vi "Adaptive Filter 2 Test.vi"(4 "Beta":fxp<+/-,32,-16>, 6 "Noise":T1, 7 "Filter Size":i32, 8 "Taps In":refnum<data-value>, 9 "Weights In":refnum<data-value>, 11 "Input":fxp<+/-,16,16>) -> (0 "Taps Out":refnum<data-value>, 1 "Weights Out":refnum<data-value>, 3 "Error Out":fxp<+/-,16,16> format="%.16g")   [LabVIEW 2016]
uses:
  <vilib>/Platform/TimedLoop/XDataNode/timing_clust.ctl
  <vilib>/Platform/TimedLoop/XDataNode/nitl_modes.ctl
  <vilib>/Platform/TimedLoop/XDataNode/wakeup.ctl
  <vilib>/Platform/TimedLoop/XDataNode/XDataNode.xnode
  <vilib>/Platform/TimedLoop/XDataNode/XDNodeRunTimeDep.lvlib
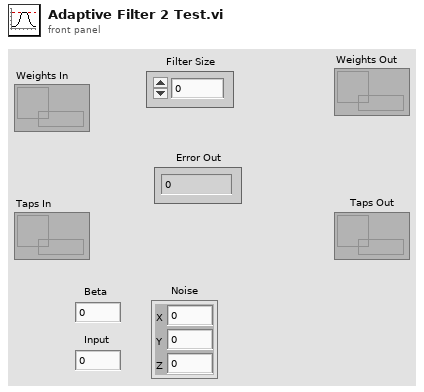
[diagram p1: front panel]
types:
  T1 = cluster{"X":fxp<+/-,16,16>, "Y":fxp<+/-,16,16>, "Z":fxp<+/-,16,16>}
  T2 = typedef "XDNodeRunTimeDep.lvlib/timing_clust.ctl" = cluster{"Expected End [f-1]":u64, "Actual End [f-1]":u64, "Finished Late? [f-1]":bool, "Expected End [i-1]":u64, "Actual End [i-1]":u64, "Finished Late? [i-1]":bool, "Expected Start [i]":u64, "Actual Start [i]":u64, "Expected Start [f]":u64, "Actual Start [f]":u64, "Source Name":string, "Structure Name":string, "Period":i64, "Deadline":i64, "Offset":i64, "Start":i64, "Priority":i32, "Timeout":i32, "Mode":T3, "Wakeup Reason":T4, "Error":errorcluster, "Source Type":string, "Secondary Source Type":string, "Global End Time":u64, "Global Start Time":u64, "Frame Duration":u64, "Iteration Duration":u64, "Assigned CPU":i32, "I/O Scan Engine Mode":u32}
  T3 = typedef "XDNodeRunTimeDep.lvlib/nitl_modes.ctl" = enum32{"No Change", "Process missed periods, maintain original phase", "Discard missed periods, maintain original phase", "Process missed periods, ignore original phase", "Discard missed periods, ignore original phase"}
  T4 = typedef "XDNodeRunTimeDep.lvlib/wakeup.ctl" = enum32{"Normal", "Aborted", "Asynchronous wakeup", "Timing source error", "Timed loop error", "Timeout"}
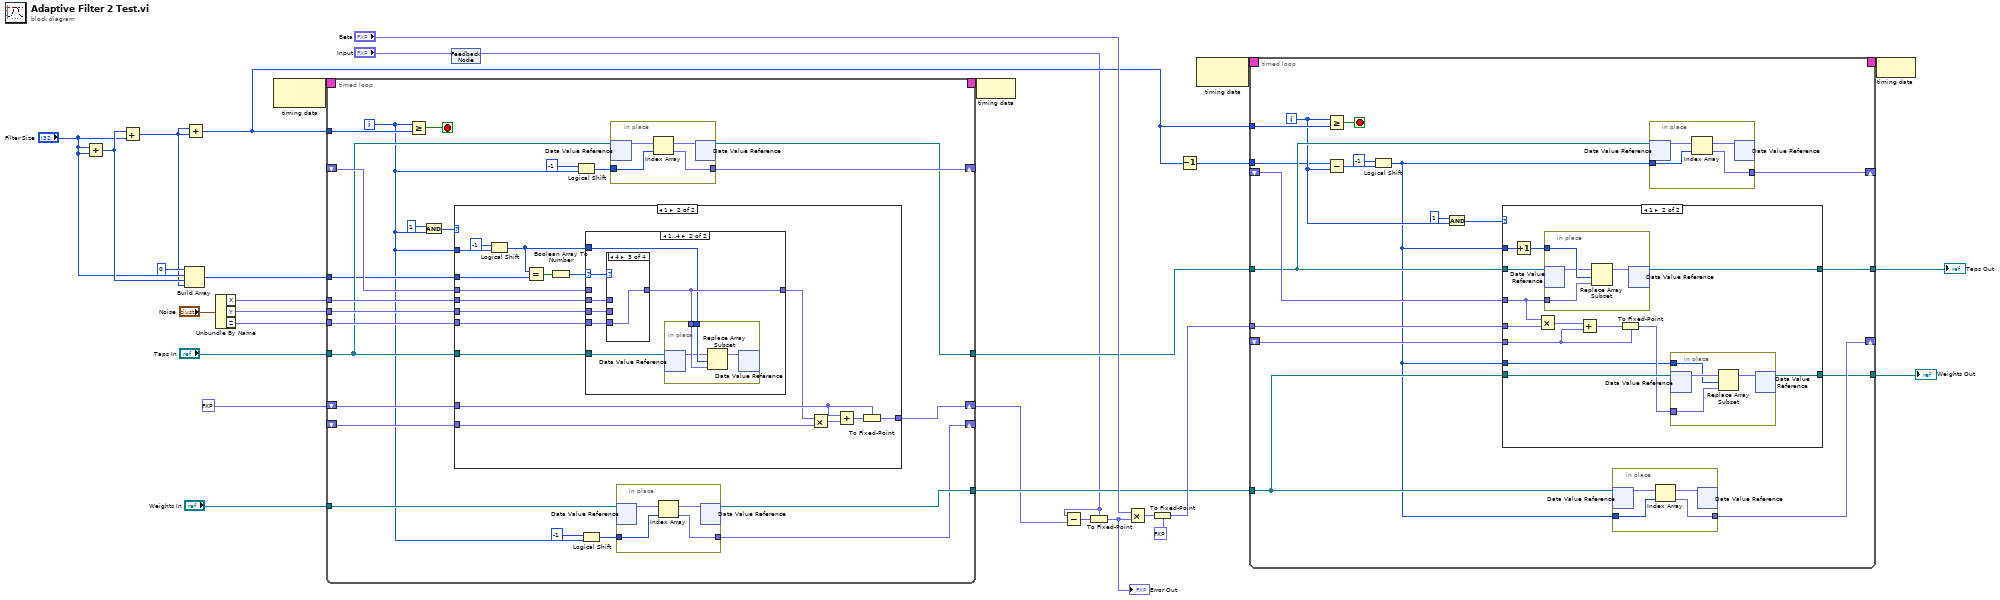
[diagram p0: block diagram]
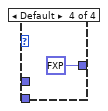
[diagram p7: hidden frame]
diagram:
  n1 = Add(x="Filter Size", y="Filter Size") -> (x+y=w12:i32)
  n2 = Add(x=w12, y="Filter Size") -> (x+y=w8:i32)
  n3 = Build Array(0 ("element"), "Filter Size", w12, w8) -> (w9:i32[])
  n4 = Add(x=w8, y=w8) -> (x+y=w6:i32)
  n5 = Unbundle By Name("Noise") -> ("X"=w30:fxp<+/-,16,16>, "Y"=w29:fxp<+/-,16,16>, "Z"=w28:fxp<+/-,16,16>)
  n6 = node-c288() -> (w24:T2)  [unwired: 1 in]
  n7 = timed-loop {
    tunnel: w30 -> [w40]
    tunnel: w29 -> [w39]
    tunnel: w28 -> [w38]
    shift-right: [w42] -> w14
    shift-left: fxp<+/-,33,19> 0.0 ("x+y") -> [w43]
    timing: w24 -> [_]
    timing-out: [_] -> w23
    tunnel: w6 -> [w53]
    tunnel: "Taps In" -> [w37]
    tunnel: "Weights In" -> [w41]
    tunnel: [w52] -> w19
    shift-right: [w51] -> _
    shift-left: _ -> [w45]
    shift-right: [w50] -> _
    shift-left: _ -> [w44]
    tunnel: [w32] -> w7
    tunnel: w9 -> [w34]
    i -> [w33]
    stop <- w54 stop-if-true
    n8 = Greater Or Equal?(x=w33, y=w53) -> (x >= y?=w54:bool)
    n9 = And(x=1 ("y"), y=w33) -> (x .and. y?=w47:i32)
    n10 = case shown="1" w47 {
      tunnel: w45 -> [_ w66]
      tunnel: w44 -> [_ w70]
      tunnel: w43 -> [w55 w69]
      tunnel: [w55 w68] -> w42
      tunnel: w40 -> [_ w64]
      tunnel: w39 -> [_ w63]
      tunnel: w38 -> [_ w62]
      tunnel: w37 -> [_ w65]
      tunnel: w34 -> [_ w61]
      tunnel: w33 -> [_ w57]
      frame 0, Default {
      }
      frame 1 {
        n11 = Logical Shift(y=i16 -1, x=w57) -> (x << y=w56:i32)
        n12 = Equal?(x=w56, y=w61) -> (x = y?=w60:bool[])
        n13 = Boolean Array To Number(Boolean array=w60) -> (number=w59:u8)
        n14 = case shown="1..4" w59 {
          selector: w59 -> [_ w79]
          tunnel: [w73 w80] -> w67
          tunnel: w66 -> [w73 _]
          tunnel: w65 -> [_ w78]
          tunnel: w64 -> [_ w77]
          tunnel: w63 -> [_ w76]
          tunnel: w62 -> [_ w75]
          tunnel: w56 -> [_ w74]
          frame Default {
          }
          frame 1..4 {
            n15 = case shown="4" w79 {
              tunnel: [w81 w82 w83 fxp<+/-,16,16> 0.0 ("Z")] -> w80
              tunnel: w77 -> [w81 _ _ _]
              tunnel: w76 -> [_ w82 _ _]
              tunnel: w75 -> [_ _ w83 _]
              frame 1 {
              }
              frame 2 {
              }
              frame 4 {
              }
              frame Default {
              }
            }
            n16 = in-place {
              in-place-border: w74 -> [w88]
              in-place-border: w80 -> [w87]
              n17 = in-place-dvr #1(w78) -> (w86:fxp<+/-,16,16>[])  [unwired: 1 out]
              n18 = Replace Array Subset(array=w86, new element=w87, index=w88) -> (w85:fxp<+/-,16,16>[])
              n19 = in-place-dvr #1(w85) -> ()  [unwired: 2 out]
            }
          }
        }
        n20 = Multiply(x=w67, y=w70) -> (x*y=w72:fxp<+/-,40,24>)
        n21 = Add(x=w69, y=w72) -> (x+y=w71:fxp<+/-,40,24>)
        n22 = To Fixed-Point(fixed-point type=w69, number=w71) -> (fixed-point=w68:fxp<+/-,33,19>)
      }
    }
    n23 = Logical Shift(y=i16 -1, x=w33) -> (x << y=w48:i32)
    n24 = Logical Shift(y=i16 -1, x=w33) -> (x << y=w35:i32)
    n25 = in-place {
      in-place-border: w48 -> [w90]
      in-place-border: [w89] -> w51
      n26 = in-place-dvr #2(w37) -> (w91:fxp<+/-,16,16>[])  [unwired: 1 out]
      n27 = Index Array(array=w91, index=w90) -> (element=w89:fxp<+/-,16,16>)
      n28 = in-place-dvr #2(w91) -> (w32:refnum<data-value>)  [unwired: 1 out]
    }
    n29 = in-place {
      in-place-border: w35 -> [w93]
      in-place-border: [w92] -> w50
      n30 = in-place-dvr #3(w41) -> (w94:fxp<+/-,24,8>[])  [unwired: 1 out]
      n31 = Index Array(array=w94, index=w93) -> (element=w92:fxp<+/-,24,8>)
      n32 = in-place-dvr #3(w94) -> (w52:refnum<data-value>)  [unwired: 1 out]
    }
  }
  n33 = feedback-in #4("Input") -> ()
  n34 = feedback #4() -> (w1:fxp<+/-,16,16>)  [unwired: 1 in]
  n35 = node-c288(w23) -> ()
  n36 = Subtract(x=w1, y=w14) -> (x-y=w27:fxp<+/-,34,20>)
  n37 = To Fixed-Point(fixed-point type=w1, number=w27) -> (fixed-point=w15:fxp<+/-,16,16>)
  "Error Out" <- w15
  n38 = Multiply(x="Beta", y=w15) -> (x*y=w26:fxp<+/-,48,0>)
  n39 = To Fixed-Point(fixed-point type=fxp<+/-,32,-1> 0.0 ("Z"), number=w26) -> (fixed-point=w25:fxp<+/-,32,-1>)
  n40 = Decrement(x=w6) -> (x-1=w5:i32)
  n41 = node-c288() -> (w22:T2)  [unwired: 1 in]
  n42 = timed-loop {
    tunnel: w25 -> [w107]
    timing: w22 -> [_]
    timing-out: [_] -> w21
    tunnel: w6 -> [w101]
    shift-right: [w111] -> _
    shift-left: _ -> [w114]
    shift-right: [w105] -> _
    shift-left: _ -> [w106]
    tunnel: w19 -> [w104]
    tunnel: [w112] -> w18
    tunnel: [w103] -> w3
    tunnel: w7 -> [w102]
    tunnel: w5 -> [w97]
    i -> [w99]
    stop <- w113 stop-if-true
    n43 = Greater Or Equal?(x=w99, y=w101) -> (x >= y?=w113:bool)
    n44 = Subtract(x=w97, y=w99) -> (x-y=w100:i32)
    n45 = Logical Shift(y=i16 -1, x=w100) -> (x << y=w98:i32)
    n46 = And(x=1, y=w99) -> (x .and. y?=w110:i32)
    n47 = case shown="1" w110 {
      tunnel: w114 -> [_ w132]
      tunnel: [w122 w135] -> w112
      tunnel: w102 -> [w122 w134]
      tunnel: w107 -> [_ w133]
      tunnel: w106 -> [_ w129]
      tunnel: w104 -> [w121 w128]
      tunnel: [w121 w127] -> w103
      tunnel: w98 -> [_ w123]
      tunnel: w98 -> [_ w125]
      frame Default {
      }
      frame 1 {
        n48 = Increment(x=w125) -> (x+1=w124:i32)
        n49 = Multiply(x=w132, y=w133) -> (x*y=w131:fxp<+/-,48,15>)
        n50 = in-place {
          in-place-border: w124 -> [w143]
          in-place-border: w132 -> [w142]
          n51 = in-place-dvr #5(w134) -> (w141:fxp<+/-,16,16>[])  [unwired: 1 out]
          n52 = Replace Array Subset(array=w141, new element=w142, index=w143) -> (w140:fxp<+/-,16,16>[])
          n53 = in-place-dvr #5(w140) -> (w135:refnum<data-value>)  [unwired: 1 out]
        }
        n54 = Add(x=w131, y=w129) -> (x+y=w130:fxp<+/-,48,15>)
        n55 = To Fixed-Point(fixed-point type=w129, number=w130) -> (fixed-point=w126:fxp<+/-,24,8>)
        n56 = in-place {
          in-place-border: w123 -> [w138]
          in-place-border: w126 -> [w137]
          n57 = in-place-dvr #6(w128) -> (w139:fxp<+/-,24,8>[])  [unwired: 1 out]
          n58 = Replace Array Subset(array=w139, new element=w137, index=w138) -> (w136:fxp<+/-,24,8>[])
          n59 = in-place-dvr #6(w136) -> (w127:refnum<data-value>)  [unwired: 1 out]
        }
      }
    }
    n60 = in-place {
      in-place-border: [w116] -> w105
      in-place-border: w98 -> [w115]
      n61 = in-place-dvr #7(w104) -> (w117:fxp<+/-,24,8>[])  [unwired: 1 out]
      n62 = Index Array(array=w117, index=w115) -> (element=w116:fxp<+/-,24,8>)
      n63 = in-place-dvr #7(w117) -> ()  [unwired: 2 out]
    }
    n64 = in-place {
      in-place-border: w98 -> [w120]
      in-place-border: [w119] -> w111
      n65 = in-place-dvr #8(w102) -> (w118:fxp<+/-,16,16>[])  [unwired: 1 out]
      n66 = Index Array(array=w118, index=w120) -> (element=w119:fxp<+/-,16,16>)
      n67 = in-place-dvr #8(w118) -> ()  [unwired: 2 out]
    }
  }
  "Taps Out" <- w18
  "Weights Out" <- w3
  n68 = node-c288(w21) -> ()
